vi "Update Movables.vi"(7 "Movables in":refnum<class "Movable.lvclass">[](array[class]), 11 "AI Manager in":refnum<class "AI Manager.lvclass">) -> (3 "AI Manager out":refnum<class "AI Manager.lvclass">)   [LabVIEW 2024, in "AI Manager.lvclass"]
doc: "MIT Licence\nCopyright (c) 2024 David Grollier"
uses:
  AI Manager.lvclass
  Game Componants/Game Board Component/Movable/Movable.lvclass
  AI Manager.lvclass/AI Manager.ctl
  Game Componants/Game Board Component/Movable/Flying Saucer/Flying Saucer.lvclass
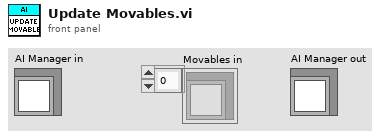
[diagram p1: front panel]
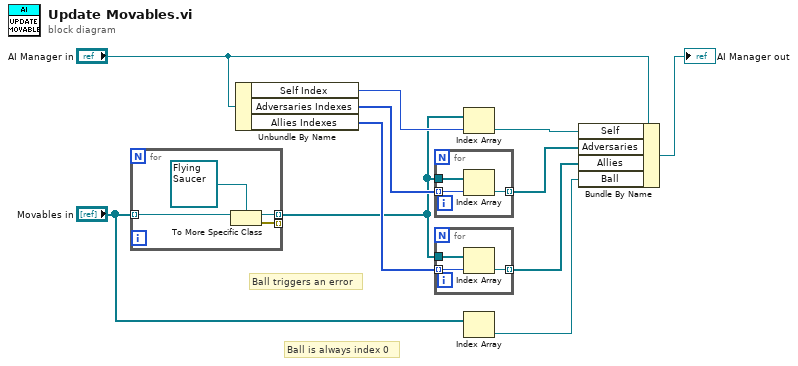
[diagram p0: block diagram]
diagram:
  # "Ball triggers an error"
  # "Ball is always index 0"
  n1 = for {
    tunnel: "Movables in" -> [w14] mode=indexing
    tunnel: [w13] -> w2 mode=indexing
    tunnel: [w12] -> _ mode=indexing
    n2 = To More Specific Class(target class=refnum<class "Flying Saucer.lvclass"> refnum ("Flying Saucer.lvclass"), reference=w14) -> (specific class reference=w13:refnum<class "Flying Saucer.lvclass">, error out=w12:errorcluster)  [unwired: 1 in]
  }
  n3 = Unbundle By Name("AI Manager in") -> ("Self Index"=w4:i32, "Adversaries Indexes"=w8:i32[], "Allies Indexes"=w6:i32[])
  n4 = for {
    tunnel: w2 -> [w18]
    tunnel: w8 -> [w17] mode=indexing
    tunnel: [w16] -> w7 mode=indexing
    n5 = Index Array(array=w18, index=w17) -> (element=w16:refnum<class "Flying Saucer.lvclass">)
  }
  n6 = for {
    tunnel: w2 -> [w21]
    tunnel: w6 -> [w20] mode=indexing
    tunnel: [w19] -> w5 mode=indexing
    n7 = Index Array(array=w21, index=w20) -> (element=w19:refnum<class "Flying Saucer.lvclass">)
  }
  n8 = Index Array(array=w2, index=w4) -> (element=w9:refnum<class "Flying Saucer.lvclass">)
  n9 = Index Array(array="Movables in") -> (element=w1:refnum<class "Movable.lvclass">)  [unwired: 1 in]
  n10 = Bundle By Name(cluster="AI Manager in", "Self"=w9, "Adversaries"=w7, "Allies"=w5, "Ball"=w1) -> (→"AI Manager out":refnum<class "AI Manager.lvclass">)
